vi "DataTransC2M.vi"(1 "input":dbl) -> (0 "output":string)   [LabVIEW 2016]
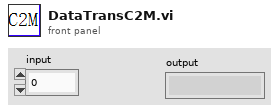
[diagram p1: front panel]
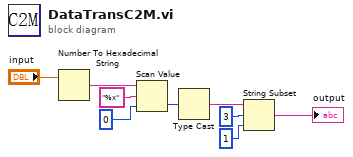
[diagram p0: block diagram]
diagram:
  n1 = Number To Hexadecimal String(2:"input") -> (0:w8:string)  [unwired: 1 in]
  n2 = Scan Value(string=w8, format string="%x", default (0 dbl)=0) -> (value=w6:i32)  [unwired: 1 out]
  n3 = Type Cast(x=w6) -> (*(type *) &x=w5:string)  [unwired: 1 in]
  n4 = String Subset(string=w5, offset (0)=3, length (rest)=1 ("length (rest)")) -> (substring=→"output":string)
